vi "Send RefreshTime Notifier.vi"(8 "error in (no error)":errorcluster, 10 "RefreshTime (ms)":u32, 11 "Transport in":refnum<class "Transport.lvclass">) -> (0 "error out":errorcluster, 3 "Transport out":refnum<class "Transport.lvclass">)   [LabVIEW 2019, in "Transport.lvclass"]
uses:
  Transport.lvclass
  Transport.lvclass/Transport.ctl
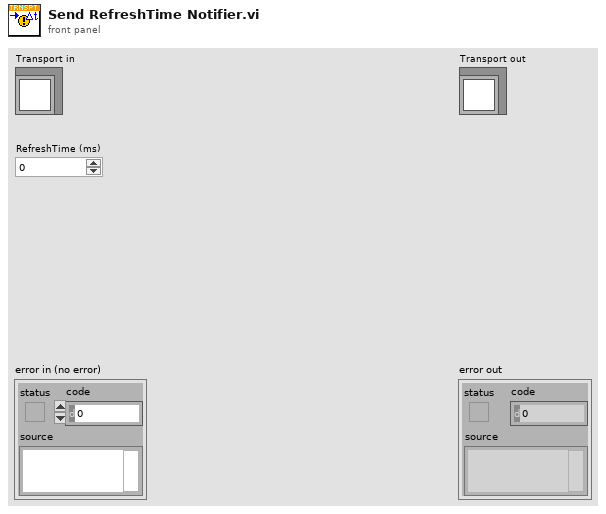
[diagram p1: front panel]
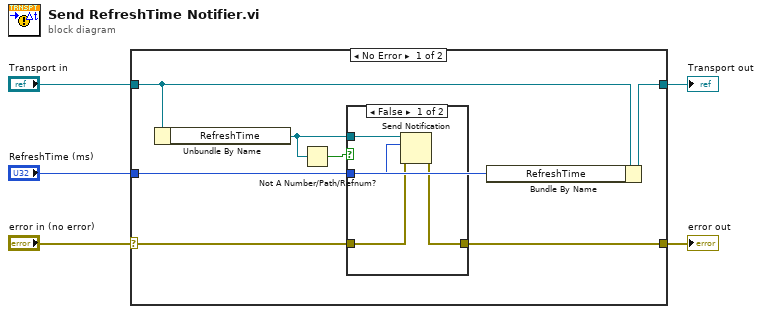
[diagram p0: block diagram]
diagram:
  n1 = case shown="No Error" "error in (no error)" {
    selector: "error in (no error)" -> [w10 w18]
    tunnel: [w9 w18] -> w4
    tunnel: [w12 w19] -> w2
    tunnel: "Transport in" -> [w11 w19]
    tunnel: "RefreshTime (ms)" -> [w8 _]
    frame No Error {
      n2 = Unbundle By Name(w11) -> ("RefreshTime"=w6:refnum<notifier>)
      n3 = Not A Number/Path/Refnum?(number/path/refnum=w6) -> (NaN/Path/Refnum?=w7:bool)
      n4 = case shown="False" w7 {
        tunnel: w6 -> [w16 _]
        tunnel: w10 -> [w15 w17]
        tunnel: [w14 w17] -> w9
        tunnel: w8 -> [w13 _]
        frame False {
          n5 = Send Notification(notification=w13, notifier=w16, error in (no error)=w15) -> (error out=w14:errorcluster)  [unwired: 1 out]
        }
        frame True {
        }
      }
      n6 = Bundle By Name(cluster=w11, "RefreshTime"=w8) -> (w12:refnum<class "Transport.lvclass">)
    }
    frame Error {
    }
  }
  "error out" <- w4
  "Transport out" <- w2
